vi "Valid.vi"(11 "Nav Route in":refnum<class "Nav Route.lvclass">) -> (2 "Valid":bool, 3 "Nav Route out":refnum<class "Nav Route.lvclass">)   [LabVIEW 2020, in "Volatus.lvlib" / "Nav Route.lvclass"]
uses:
  Nav Route.lvclass
  Nav Route.lvclass/Nav Route.ctl
  lv-exec-anchor/ExecAnchor/ExecAnchor.lvclass
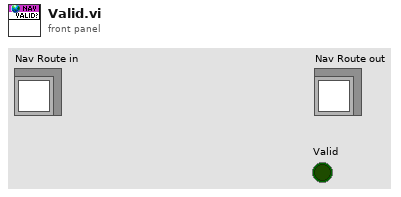
[diagram p1: front panel]
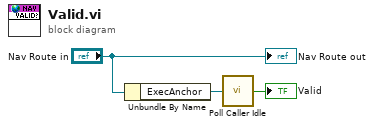
[diagram p0: block diagram]
diagram:
  n1 = Unbundle By Name("Nav Route in") -> ("ExecAnchor"=w2:refnum<class "ExecAnchor.lvclass">)
  n2 = call "Poll Caller Idle.vi"("ExecAnchor in"=w2) -> ("Caller Idle"=→"Valid":bool)  [unwired: 3 in, 1 out]
  "Nav Route out" <- "Nav Route in"
